vi "Analyse_day_files.vi"() -> ()   [LabVIEW 2020]
panel:
  out "Night Total":dbl
  in  "Path name in":path
  out "Day Total KWHrs":dbl
  in  "Today":bool=TRUE
  out "Second taken":dbl format="%.2f"
  in  "Data folder location":path
  in  "End Date":T1={"day of month"=0, "month"=0, "year"=1999} {"year" min=1998 max=2100}
  in  "Start Date":T1={"day of month"=0, "month"=0, "year"=1999} {"year" min=1998 max=2100}
  out "Plot":cluster{dbl[], dbl[]}(graph)
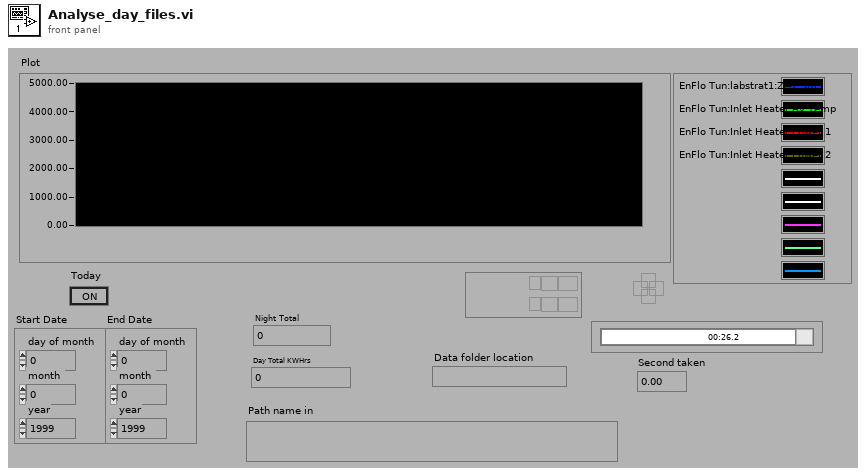
[diagram p1: front panel]
types:
  T1 = cluster{"day of month":i32, "month":i32, "year":i32}
  T2 = cluster{"second":i32, "minute":i32, "hour":i32, "day of month":i32, "month":i32, "year":i32, "day of week":i32, "day of year":i32, "is DST":i32}
  T3 = cluster{"day of month":i32, "month":i32, "year":i32}[]
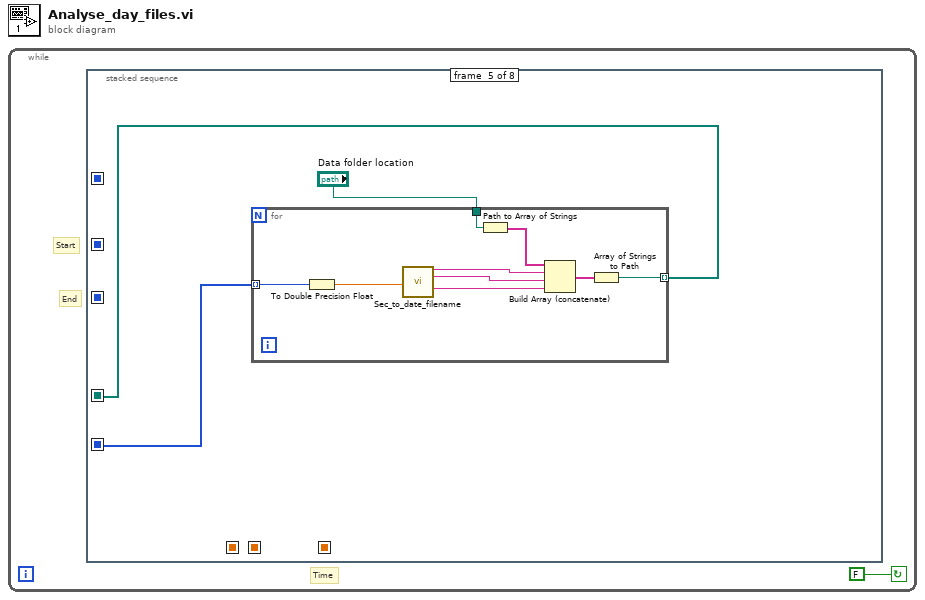
[diagram p0: block diagram]
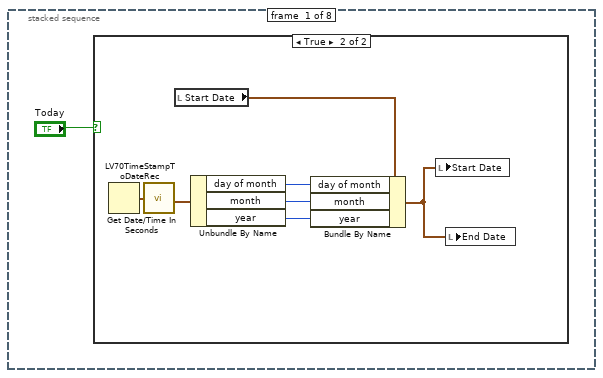
[diagram p2: hidden frame]
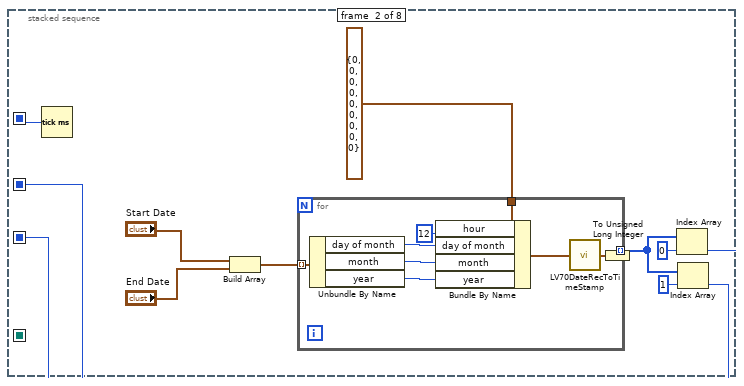
[diagram p4: hidden frame]
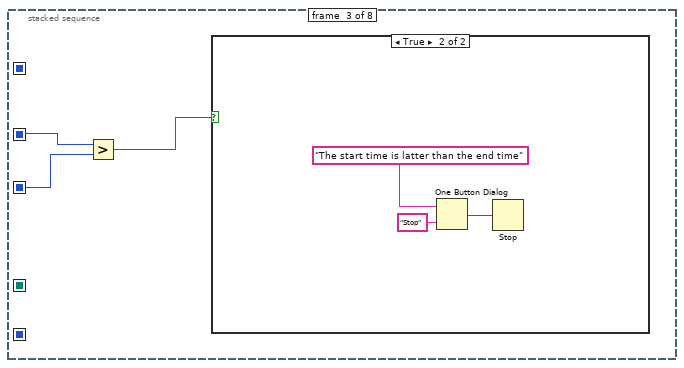
[diagram p5: hidden frame]
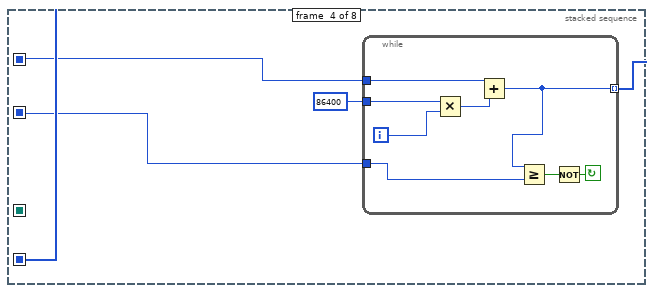
[diagram p7: hidden frame]
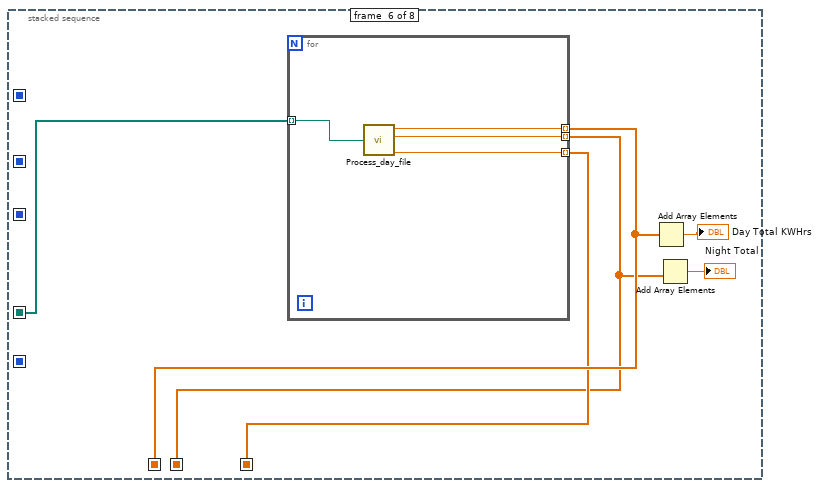
[diagram p8: hidden frame]
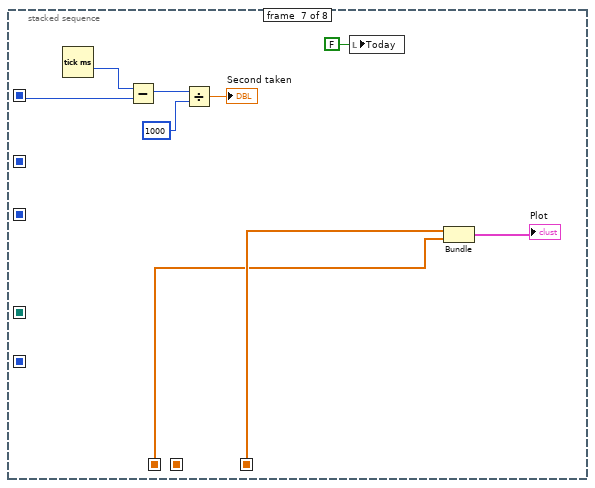
[diagram p9: hidden frame]
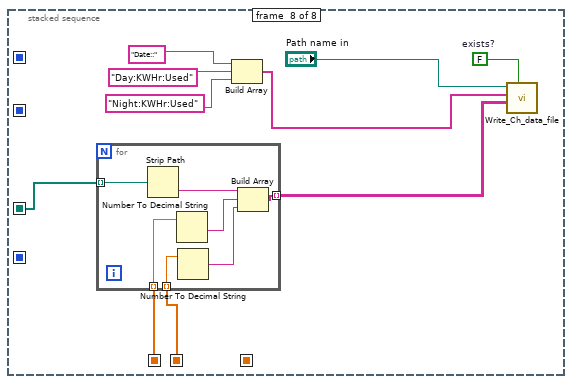
[diagram p10: hidden frame]
diagram:
  n1 = while {
    stop <- FALSE continue-if-true
    # "Time"
    # "End"
    # "Start"
    n2 = stacked-sequence {
      seq-local: [_ _ _ w38 _ _ _ _] -> [_ _ _ _ w49 _ _ _]
      seq-local: [_ _ _ _ w48 _ _ _] -> [_ _ _ _ _ w64 _ w87]
      seq-local: [_ _ _ _ _ w62 _ _] -> [_ _ _ _ _ _ w69 w83]
      seq-local: [_ _ _ _ _ w60 _ _] -> [_ _ _ _ _ _ w70 _]
      seq-local: [_ w14 _ _ _ _ _ _] -> [_ _ w30 w37 _ _ _ _]
      seq-local: [_ w13 _ _ _ _ _ _] -> [_ _ w31 w36 _ _ _ _]
      seq-local: [_ w11 _ _ _ _ _ _] -> [_ _ _ _ _ _ w76 _]
      seq-local: [_ _ _ _ _ w59 _ _] -> [_ _ _ _ _ _ _ w80]
      frame #0 {
        n3 = case shown="True" "Today" {
          frame False {
          }
          frame True {
            n4 = Get Date/Time In Seconds() -> (seconds since 1Jan1904=w3:timestamp)
            n5 = call <vilib>:"LV70TimeStampToDateRec.vi"("time stamp"=w3) -> ("date time rec"=w9:T2)
            n6 = local read "Start Date"() -> (w8:T1)
            n7 = Unbundle By Name(w9) -> ("day of month"=w7:i32, "month"=w6:i32, "year"=w5:i32)
            n8 = Bundle By Name(cluster=w8, "day of month"=w7, "month"=w6, "year"=w5) -> (w4:T1)
            n9 = local write "Start Date"(w4) -> ()
            n10 = local write "End Date"(w4) -> ()
          }
        }
      }
      frame #1 {
        n11 = Tick Count (ms)() -> (millisecond timer value=w11:u32)
        n12 = Build Array("Start Date", "End Date") -> (w17:T3)
        n13 = for {
          tunnel: T2 {"second"=0, "minute"=0, "hour"=0, "day of month"=0, "month"=0, "year"=0, "day of week"=0, "day of year"=0, "is DST"=0} ("date time rec") -> [w28]
          tunnel: w17 -> [w22] mode=indexing
          tunnel: [w21] -> w12 mode=indexing
          n14 = Unbundle By Name(w22) -> ("day of month"=w27:i32, "month"=w26:i32, "year"=w25:i32)
          n15 = Bundle By Name(cluster=w28, "hour"=12, "day of month"=w27, "month"=w26, "year"=w25) -> (w23:T2)
          n16 = call <vilib>:"LV70DateRecToTimeStamp.vi"("date time rec"=w23) -> ("Time Stamp"=w20:timestamp)
          n17 = To Unsigned Long Integer(number=w20) -> (unsigned 32bit integer=w21:u32)
        }
        n18 = Index Array(array=w12, index=0) -> (element=w14:u32)
        n19 = Index Array(array=w12, index=1) -> (element=w13:u32)
      }
      frame #2 {
        n20 = Greater?(x=w30, y=w31) -> (0:w29:bool)
        n21 = case shown="True" w29 {
          frame False {
          }
          frame True {
            n22 = One Button Dialog(message="The start time is latter than the end time", button name ("OK")="Stop") -> (true=w33:bool)
            n23 = Stop(stop? (T)=w33) -> ()
          }
        }
      }
      frame #3 {
        n24 = while {
          tunnel: [w39] -> w38 mode=indexing
          tunnel: w36 -> [w46]
          tunnel: w37 -> [w40]
          tunnel: u32 86400 ("seconds") -> [w42]
          i -> [w43]
          stop <- w44 continue-if-true
          n25 = Multiply(x=w42, y=w43) -> (x*y=w41:u32)
          n26 = Add(x=w40, y=w41) -> (x+y=w39:u32)
          n27 = Greater Or Equal?(x=w39, y=w46) -> (x >= y?=w45:bool)
          n28 = Not(x=w45) -> (.not. x?=w44:bool)
        }
      }
      frame #4 {
        n29 = for {
          tunnel: w49 -> [w58] mode=indexing
          tunnel: "Data folder location" -> [w55]
          tunnel: [w51] -> w48 mode=indexing
          n30 = To Double Precision Float(number=w58) -> (double precision float=w57:dbl)
          n31 = call "Sec_to_date_filename.vi"("ss1904"=w57) -> ("YYYY"=w54:string, "mm-YYYY"=w50:string, "DD-mm-YYYY"=w53:string)  [unwired: 5 in, 7 out]
          n32 = Path to Array of Strings(0:w55) -> (2:w56:string[])  [unwired: 1 out]
          n33 = Build Array (concatenate)(w56, w54, w50, w53) -> (w52:string[])
          n34 = Array of Strings to Path(0:w52) -> (2:w51:path)  [unwired: 1 out]
        }
      }
      frame #5 {
        n35 = for {
          tunnel: w64 -> [w68] mode=indexing
          tunnel: [w67] -> w62 mode=indexing
          tunnel: [w66] -> w59 mode=indexing
          tunnel: [w65] -> w60 mode=indexing
          n36 = call "Process_day_file.vi"("Filename"=w68) -> ("Day KW Hrs"=w67:dbl, "Night KWHrs"=w66:dbl, "Time"=w65:dbl)  [unwired: 7 out]
        }
        n37 = Add Array Elements(numeric array=w62) -> (sum=→"Day Total KWHrs":dbl)
        n38 = Add Array Elements(numeric array=w59) -> (sum=→"Night Total":dbl)
      }
      frame #6 {
        n39 = Tick Count (ms)() -> (millisecond timer value=w77:u32)
        n40 = Subtract(x=w77, y=w76) -> (x-y=w75:u32)
        n41 = Divide(x=w75, y=u32 1000) -> (x/y=→"Second taken":dbl)
        n42 = local write "Today"(FALSE ("Today")) -> ()
        n43 = Bundle(w70, w69) -> (→"Plot":cluster{dbl[], dbl[]})  [unwired: 1 out]
      }
      frame #7 {
        w81 = FALSE  # exists?
        n44 = for {
          tunnel: w87 -> [w94] mode=indexing
          tunnel: w83 -> [w93] mode=indexing
          tunnel: [w90] -> w82 mode=indexing
          tunnel: w80 -> [w89] mode=indexing
          n45 = Strip Path(path=w94) -> (name=w92:string)  [unwired: 1 out]
          n46 = Number To Decimal String(number=w93) -> (decimal integer string=w91:string)  [unwired: 1 out]
          n47 = Number To Decimal String(number=w89) -> (decimal integer string=w88:string)  [unwired: 1 out]
          n48 = Build Array(w92, w91, w88) -> (w90:string[])
        }
        n49 = Build Array("Date::", "Day:KWHr:Used", "Night:KWHr:Used") -> (w84:string[])
        n50 = call "Write_Ch_data_file.vi"("exists?"=w81, "Channel Values"=w82, "Channel names"=w84, "Filename"="Path name in") -> ()  [unwired: 3 in, 5 out]
      }
    }
  }
